vi "MH_WritePTUHeader.vi"(8 "entrée d'erreur":errorcluster) -> (0 "sortie d'erreur":errorcluster, 3 "refnum Out":refnum<file>)   [LabVIEW 2019]
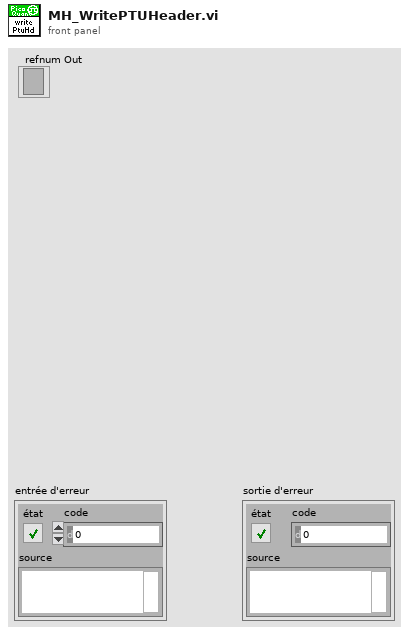
[diagram p1: front panel]
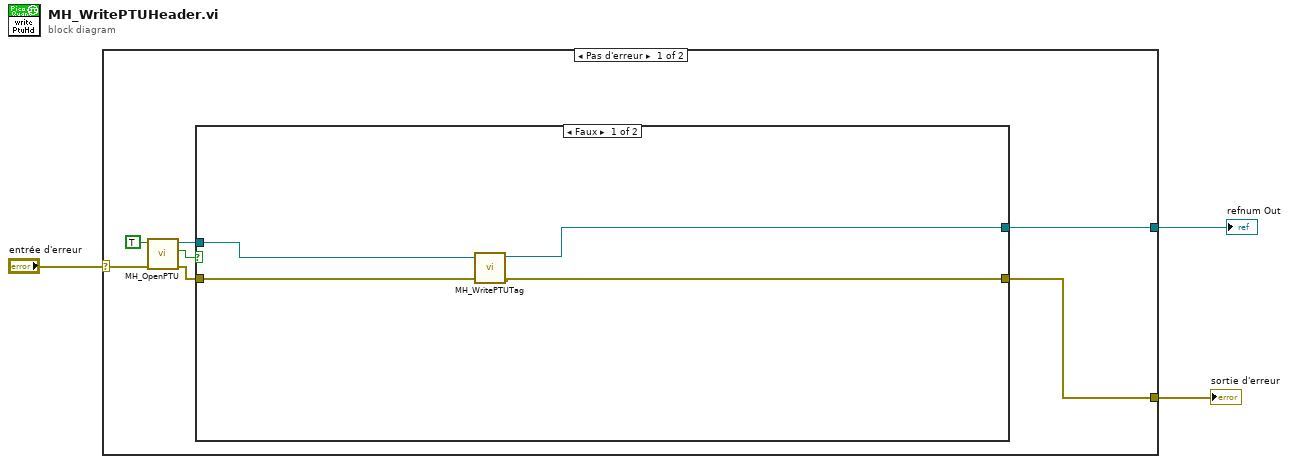
[diagram p0: block diagram]
diagram:
  n1 = case shown="Pas d'erreur" "entrée d'erreur" {
    selector: "entrée d'erreur" -> [w5 w16]
    tunnel: [w10 w16] -> w3
    tunnel: [w9 _] -> w1
    frame No Error {
      n2 = call <userlib>:"MH_OpenPTU.vi"("entrée d'erreur"=w5, "WriteMode"=TRUE) -> ("sortie d'erreur"=w6:errorcluster, "Cancelled"=w7:bool, "refnum en sortie"=w8:refnum<file>)  [unwired: 7 in]
      n3 = case shown="Faux" w7 {
        tunnel: w6 -> [w14 w15]
        tunnel: [w11 w15] -> w10
        tunnel: [w12 _] -> w9
        tunnel: w8 -> [w13 _]
        frame False {
          n4 = call <userlib>:"MH_WritePTUTag.vi"("refnum"=w13, "error in"=w14) -> ("refnum en sortie"=w12:refnum<file>, "error out"=w11:errorcluster)  [unwired: 7 in]
        }
        frame True {
        }
      }
    }
    frame Error {
    }
  }
  "sortie d'erreur" <- w3
  "refnum Out" <- w1
